vi "CheckEndStop.vi"() -> ()   [LabVIEW 2021]
uses:
  <vilib>/MakerHub/LINX/Public/Peripherals/Digital/Digital Read 1 Chan.vi
  <vilib>/MakerHub/LINX/Public/Peripherals/Digital/Digital Read N Chans.vi
  <vilib>/MakerHub/LINX/Private/Local IO/LinxDigitalRead.vi
  <vilib>/MakerHub/LINX/Public/Utilities/Check Channel.vi
  <vilib>/MakerHub/LINX/Public/Utilities/Open Serial.vi
  <vilib>/MakerHub/LINX/Private/Utilties/Generate Error.vi
  <vilib>/MakerHub/LINX/LMH-LINX.lvlib
panel:
  in  "stop":bool
  out "error out":errorcluster
  in  "error in (no error)":errorcluster
  in  "Serial Port":refnum<visa-resource-name>="N/A"
  out "DI Value":bool
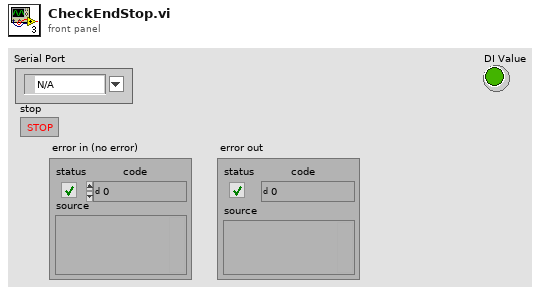
[diagram p1: front panel]
types:
  T1 = typedef "LMH-LINX.lvlib/LINX Ref.ctl" = cluster{"IO":T2, "Interface":T3, "LINX Device Config":T4}
  T2 = typedef "LMH-LINX.lvlib/Platform.ctl" = enum16{"Remote", "Local"}
  T3 = typedef "LMH-LINX.lvlib/Interface.ctl" = enum16{"Serial", "TCP"}
  T4 = typedef "LMH-LINX.lvlib/Device.lvlib/LINX Device Config.ctl" = cluster{"Interface":T3, "COM Port":refnum<visa-resource-name>, "TCP Configuration":T5, "Device Family":u8, "Device ID":u8, "Device Name":string, "TCP Ref":refnum<k5>, "Channels":T6}
  T5 = typedef "LMH-LINX.lvlib/Device.lvlib/TCP Config.ctl" = cluster{"IP Address":string, "Port":u16}
  T6 = typedef "LMH-LINX.lvlib/Channels.ctl" = cluster{"DI":u8[], "DO":u8[], "AI":u8[], "AO":u8[], "PWM":u8[], "QE":u8[], "UART":u8[], "I2C 2":u8[], "SPI":u8[], "CAN":u8[], "Servo":u8[], "AI Ref (V)":dbl, "AI Resolution (Bits)":u8, "AO Ref (V)":dbl, "AO Resolution (Bits)":u8}
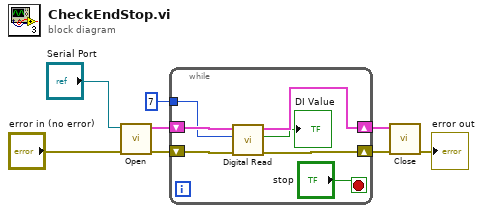
[diagram p0: block diagram]
diagram:
  n1 = call-poly <vilib>:"Open.vi"("Error In"="error in (no error)", "Serial Port"="Serial Port") -> ("Error Out"=w4:errorcluster, "LINX Resource"=w8:T1)  [unwired: 7 in, 1 out]
  n2 = while {
    tunnel: u8 7 ("DI Channel") -> [w13]
    shift-right: [w14] -> w7
    shift-left: w8 -> [w15]
    shift-right: [w10] -> w3
    shift-left: w4 -> [w11]
    stop <- "stop" stop-if-true
    n3 = call-poly <vilib>:"Digital Read.vi"("Error In"=w11, "DI Channel"=w13, "LINX Resource"=w15) -> ("Error Out"=w10:errorcluster, "DI Value"=→"DI Value":bool, "LINX Resource"=w14:T1)  [unwired: 6 in]
  }
  n4 = call <vilib>:"Close.vi"("Error In"=w3, "LINX Resource"=w7) -> ("Error Out"=→"error out":errorcluster)  [unwired: 9 in]
